vi "Launch Connection Handler.vi"(8 "error in (no error)":errorcluster, 9 "ConnectionID":i32, 10 "References in":T1, 11 "WebSocket Connection in":refnum<class "WebSocket Server.lvclass">) -> (0 "error out":errorcluster)   [LabVIEW 2019]
uses:
  <vilib>/MediaMongrels Ltd/WebSockets/WebSockets/WebSocket Server/WebSocket Server.lvclass
  <vilib>/MediaMongrels Ltd/Message Queue Helper/ctl_QMH_Message_Typedef.ctl
  <vilib>/MediaMongrels Ltd/Message Queue Helper/MessageQueueHelper.lvlib
  SubVIs/References.ctl
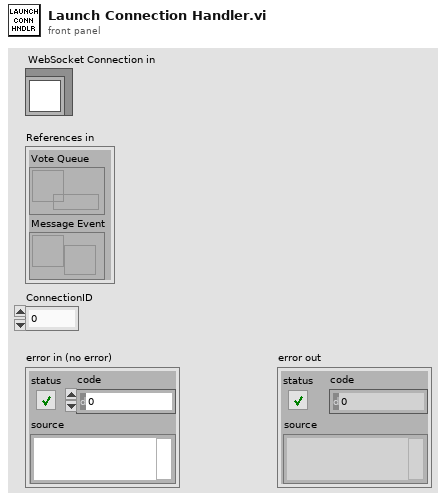
[diagram p1: front panel]
types:
  T1 = typedef "References.ctl" = cluster{"Vote Queue":refnum<queue>, "Message Event":refnum<user-event>}
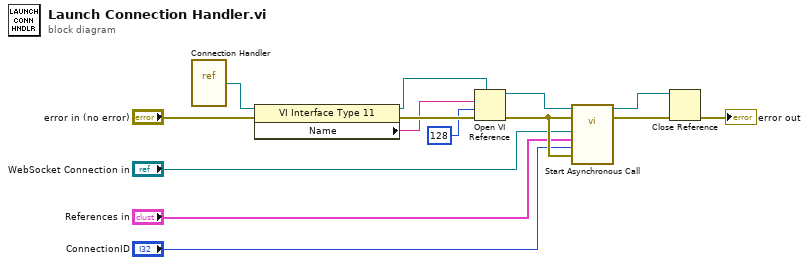
[diagram p0: block diagram]
diagram:
  n1 = vi-ref "Connection Handler.vi"() -> (w14:refnum<vi>)
  n2 = property class="VI Interface Type 11"(reference=w14, error in="error in (no error)") -> (reference out=w10:refnum<vi>, error out=w12:errorcluster, "Name"=w11:string)
  n3 = Open VI Reference(type specifier VI Refnum (for type only)=w10, vi path=w11, options=128, error in (no error)=w12) -> (vi reference=w8:refnum<vi>, error out=w4:errorcluster)  [unwired: 2 in]
  n4 = call-by-ref "Start Asynchronous Call"(reference=w8, error in=w4, 8:"error in (no error)"=w4, "ConnectionID"="ConnectionID", "References in"="References in", "WebSocket Connection in"="WebSocket Connection in") -> (reference out=w6:refnum<vi>, error out=w7:errorcluster)  [unwired: 7 in, 1 out]
  n5 = Close Reference(reference=w6, error in (no error)=w7) -> (error out=→"error out":errorcluster)
